vi "GL_Initialize.vi"(5 "IP Address/COM":string, 6 "error in (no error)":errorcluster, 9 "Galil.IGalil":refnum<k7>) -> (0 "error out":errorcluster, 1 "Connected To:":string, 2 "Library Version:":string, 3 "GL Ref Out":refnum<k7>)   [LabVIEW 2022 SP3]
doc: "Initializes the specified controller according to the settings as configured in Measurement & Automation Explorer."
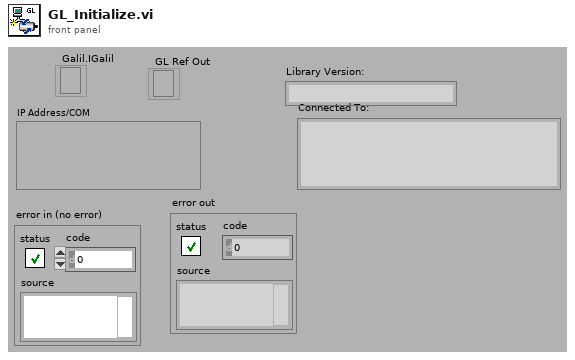
[diagram p1: front panel]
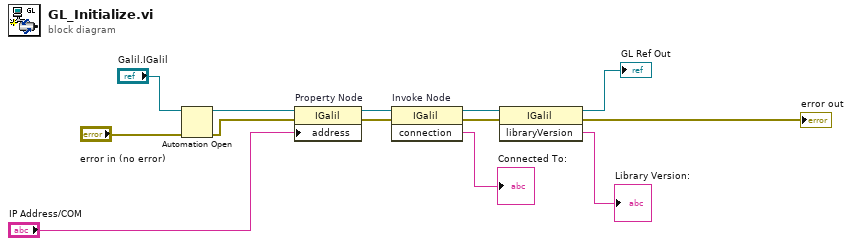
[diagram p0: block diagram]
diagram:
  n1 = Automation Open(error in (no error)="error in (no error)", Automation Refnum="Galil.IGalil") -> (Automation Refnum=w13:refnum<k7>, error out=w10:errorcluster)  [unwired: 2 out]
  n2 = property on="Property Node" class="IGalil"(reference=w13, error in=w10, "address"="IP Address/COM") -> (reference out=w12:refnum<k7>, error out=w11:errorcluster)
  n3 = invoke on="Invoke Node" class="IGalil" method="connection"(reference=w12, error in=w11) -> (reference out=w8:refnum<k7>, error out=w7:errorcluster, "connection"=→"Connected To:":string)  [unwired: 1 in]
  n4 = invoke class="IGalil" method="libraryVersion"(reference=w8, error in=w7) -> (reference out=→"GL Ref Out":refnum<k7>, error out=→"error out":errorcluster, "libraryVersion"=→"Library Version:":string)  [unwired: 1 in]
